vi "VISA Settings.vi"() -> (0 "ErrorOut":errorcluster, 2 "Path Out":path, 3 "VISA resource name out":refnum<visa-resource-name>)   [LabVIEW 2017]
uses:
  I28 Drivers/I28Drivers.lvlib
panel:
  in  "Select Log Folder Path":path
  in  "Connect":bool
  in  "BaudRate":u32=115200
  in  "VISAResourceName":refnum<visa-resource-name>
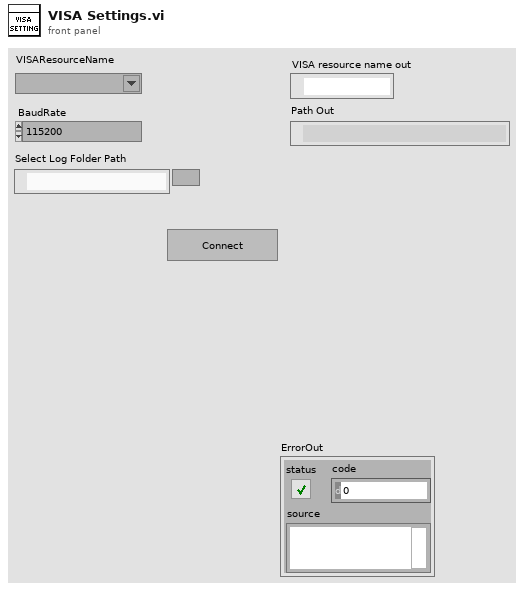
[diagram p1: front panel]
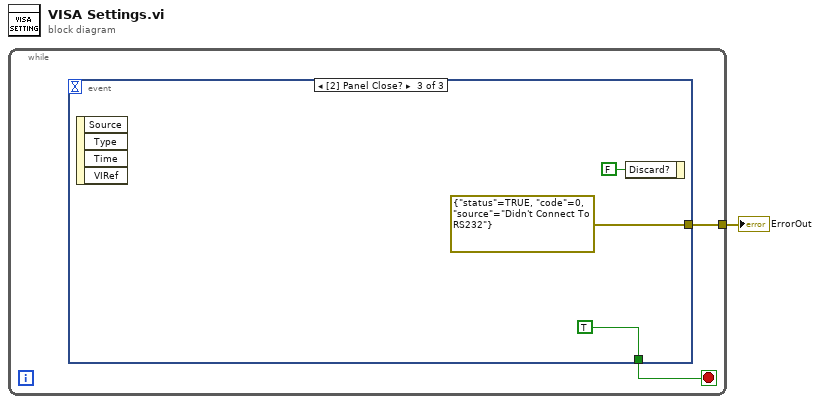
[diagram p0: block diagram]
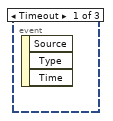
[diagram p2: hidden frame]
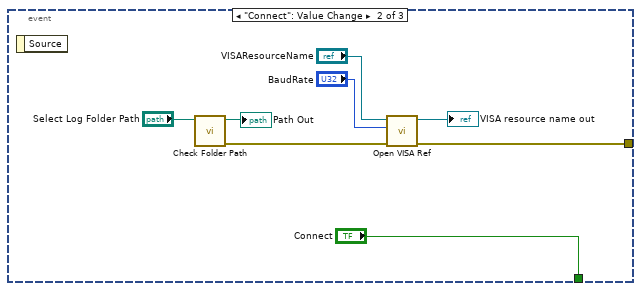
[diagram p3: hidden frame]
diagram:
  n1 = while {
    tunnel: [w2] -> w1
    stop <- w3 stop-if-true
    n2 = event shown="[2] Panel Close?" {
      selector: _ -> [_ _ _]
      dyn-events: _ -> [_ _ _]
      timeout: _ -> [_ _ _]
      tunnel: [_ "Connect" TRUE ("Connect")] -> w3
      tunnel: [_ w7 errorcluster {"status"=TRUE, "code"=0, "source"="Didn't Connect To RS232"} ("ErrorOut")] -> w2
      event Timeout {
        n3 = event-data() -> ()  [unwired: 1 in, 3 out]
      }
      event "Connect": Value Change {
        n4 = event-data() -> ()  [unwired: 1 in, 1 out]
        n5 = call "Check Folder Path.vi"("Path In"="Select Log Folder Path") -> ("error out"=w6:errorcluster, "Path Out"=→"Path Out":path)  [unwired: 9 in]
        n6 = call "Open VISA Ref.vi"("ErrorIn"=w6, "BaudRate"="BaudRate", "VISAResourceName"="VISAResourceName") -> ("ErrorOut"=w7:errorcluster, "VISA resource name out"=→"VISA resource name out":refnum<visa-resource-name>)  [unwired: 7 in]
      }
      event Panel Close? {
        n7 = event-data() -> ()  [unwired: 1 in, 4 out]
        n8 = event-data("Discard?"=FALSE) -> ()  [unwired: 1 in, 1 out]
      }
    }
  }
  "ErrorOut" <- w1
